vi "setCategoryAmount.vi"(8 "error in (no error)":errorcluster, 10 "Category.lvclass":refnum<class "Category.lvclass">, 11 "Account History in":refnum<class "Account History.lvclass">) -> (0 "error out":errorcluster, 3 "Account History out":refnum<class "Account History.lvclass">)   [LabVIEW 2018, in "Account History.lvclass"]
uses:
  Account History.lvclass
  Category/Category.lvclass
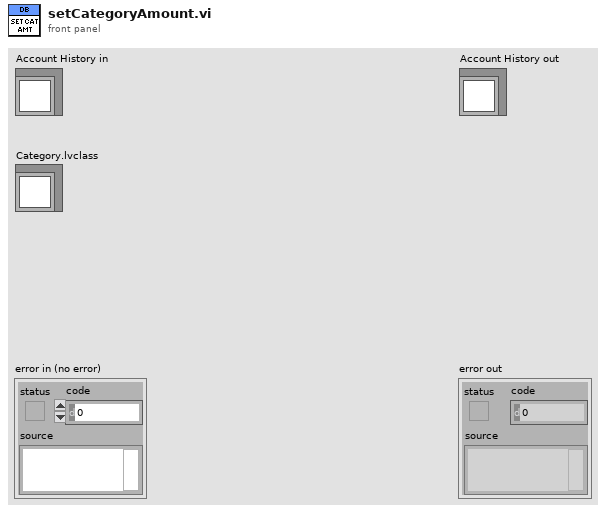
[diagram p1: front panel]
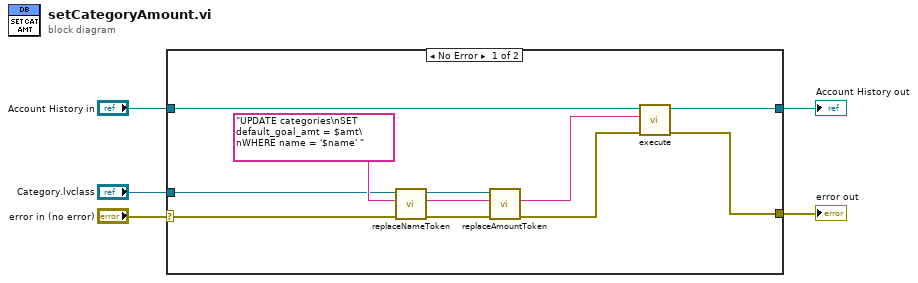
[diagram p0: block diagram]
diagram:
  n1 = case shown="No Error" "error in (no error)" {
    selector: "error in (no error)" -> [w7 w18]
    tunnel: [w14 w18] -> w4
    tunnel: [w15 w17] -> w2
    tunnel: "Account History in" -> [w16 w17]
    tunnel: "Category.lvclass" -> [w6 _]
    frame No Error {
      n2 = call "replaceNameToken.vi"("error in (no error)"=w7, "Query In"="UPDATE categories\nSET default_goal_amt = $amt\nWHERE name = '$name' ", "Category in"=w6) -> ("error out"=w12:errorcluster, "Query Out"=w10:string, "Category out"=w11:refnum<class "Category.lvclass">)  [unwired: 6 in]
      n3 = call "replaceAmountToken.vi"("error in (no error)"=w12, "Query In"=w10, "Category in"=w11) -> ("error out"=w8:errorcluster, "Query Out"=w9:string)  [unwired: 6 in, 1 out]
      n4 = call "execute.vi"("error in (no error)"=w8, "SQL query"=w9, "Database in"=w16) -> ("error out"=w14:errorcluster, "Database out"=w15:refnum<class "Account History.lvclass">)  [unwired: 7 in]
    }
    frame Error {
    }
  }
  "error out" <- w4
  "Account History out" <- w2
